vi "401_Security_Data_Convert_To_String.vi"(9 "Current Value":i32, 10 "Previous Value":i32, 11 "Label":string) -> (2 "Current Value Str":string, 3 "Previous Value Str":string)   [LabVIEW 2015]
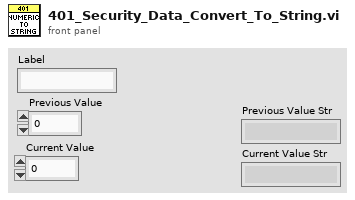
[diagram p1: front panel]
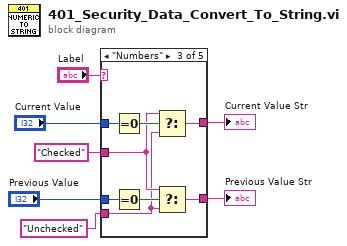
[diagram p0: block diagram]
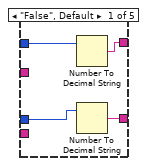
[diagram p2: hidden frame]
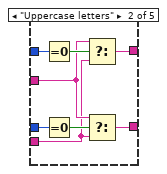
[diagram p3: hidden frame]
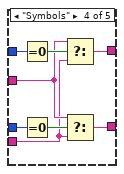
[diagram p4: hidden frame]
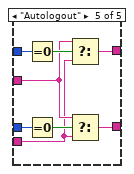
[diagram p5: hidden frame]
diagram:
  n1 = case shown="\"Numbers\"" "Label" {
    tunnel: "Checked" -> [_ w15 w23 w31 w39]
    tunnel: "Unchecked" -> [_ w14 w22 w30 w38]
    tunnel: [w10 w18 w26 w34 w42] -> w2
    tunnel: "Previous Value" -> [w11 w17 w25 w33 w41]
    tunnel: "Current Value" -> [w9 w13 w20 w29 w37]
    tunnel: [w8 w12 w21 w28 w36] -> w1
    frame "False", Default {
      n2 = Number To Decimal String(number=w9) -> (decimal integer string=w8:string)  [unwired: 1 in]
      n3 = Number To Decimal String(number=w11) -> (decimal integer string=w10:string)  [unwired: 1 in]
    }
    frame "Uppercase letters" {
      n4 = Equal To 0?(x=w13) -> (x = 0?=w16:bool)
      n5 = Equal To 0?(x=w17) -> (x = 0?=w19:bool)
      n6 = Select(t=w15, s=w16, f=w14) -> (s? t:f=w12:string)
      n7 = Select(t=w15, s=w19, f=w14) -> (s? t:f=w18:string)
    }
    frame "Numbers" {
      n8 = Equal To 0?(x=w20) -> (x = 0?=w24:bool)
      n9 = Equal To 0?(x=w25) -> (x = 0?=w27:bool)
      n10 = Select(t=w23, s=w24, f=w22) -> (s? t:f=w21:string)
      n11 = Select(t=w23, s=w27, f=w22) -> (s? t:f=w26:string)
    }
    frame "Symbols" {
      n12 = Equal To 0?(x=w29) -> (x = 0?=w32:bool)
      n13 = Equal To 0?(x=w33) -> (x = 0?=w35:bool)
      n14 = Select(t=w31, s=w32, f=w30) -> (s? t:f=w28:string)
      n15 = Select(t=w31, s=w35, f=w30) -> (s? t:f=w34:string)
    }
    frame "Autologout" {
      n16 = Equal To 0?(x=w37) -> (x = 0?=w40:bool)
      n17 = Equal To 0?(x=w41) -> (x = 0?=w43:bool)
      n18 = Select(t=w39, s=w40, f=w38) -> (s? t:f=w36:string)
      n19 = Select(t=w39, s=w43, f=w38) -> (s? t:f=w42:string)
    }
  }
  "Previous Value Str" <- w2
  "Current Value Str" <- w1
